vi "MFC R AirC1.vi"(3 "error in":errorcluster) -> (8 "MFC out":u8[](array[numeric]), 10 "error out":errorcluster)   [LabVIEW 2014]
uses:
  <vilib>/eio/EIOMethodNode/EIOMethodNode.xnode
  <vilib>/rvi/eio/common/nirviEmuTemplateMethod_errors.vi
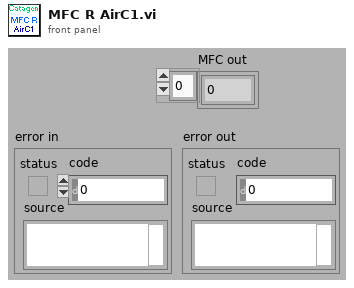
[diagram p1: front panel]
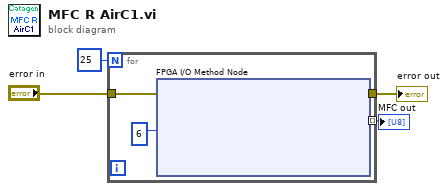
[diagram p0: block diagram]
diagram:
  n1 = for {
    N: 25 -> [_]
    tunnel: "error in" -> [w7]
    tunnel: [w6] -> w1
    tunnel: [w5] -> w2 mode=indexing
    n2 = xnode "FPGA I/O Method Node"("error in"=w7, "Timeout (ms)"=6) -> ("error out"=w6:errorcluster, "Data"=w5)  [unwired: 1 in, 2 out]
  }
  "error out" <- w1
  "MFC out" <- w2
